vi "Encoder_sub_VI.vi"(8 "error in (no error)":errorcluster) -> (0 "error out":errorcluster, 3 "Encoder Output":T1)   [LabVIEW 2017]
uses:
  Encoder Cluster.ctl
  <vilib>/myRIO/Common/Instrument Driver Framework/myRIO v1.0/Encoder/typedefs/Encoder Count Direction Enum.ctl
  <vilib>/myRIO/Common/Instrument Driver Framework/myRIO v1.0/Encoder/typedefs/Encoder Signal Mode.ctl
  <vilib>/myRIO/Instrument Drivers/Onboard IO/Encoder/typedefs/Encoder Reference.ctl
  <vilib>/myRIO/Common/Instrument Driver Framework/Utilities/typedefs/myRIO Generic Hardware Reference.ctl
  <vilib>/myRIO/Common/Instrument Driver Framework/Utilities/typedefs/Hardware Version Enum.ctl
  <vilib>/myRIO/Common/Instrument Driver Framework/Utilities/typedefs/myRIO v1.0 Reference.ctl
  <vilib>/myRIO/Common/Instrument Driver Framework/Utilities/typedefs/Generic FPGA Reference.ctl
  <vilib>/myRIO/Common/Instrument Driver Framework/myRIO v1.0/Encoder/typedefs/Encoder Channels Enum.ctl
  <vilib>/myRIO/Common/Instrument Driver Framework/myRIO v1.0/Encoder/typedefs/Encoder Configuration v1.0.ctl
  <vilib>/userdefined/High Color/nirio_resource_hc.ctl
  <vilib>/myRIO/Common/Instrument Driver Framework/Utilities/vis/Is FPGA Ref Available.vi
  <vilib>/myRIO/Common/Instrument Driver Framework/myRIO v1.0/Encoder/vis/myRIO v1.1 Open Encoder.vi
  <vilib>/myRIO/Instrument Drivers/Onboard IO/Encoder/vis/Read.vi
  <vilib>/myRIO/Common/Instrument Driver Framework/Utilities/vis/Validate Channels.vi
  <vilib>/myRIO/Common/Instrument Driver Framework/myRIO v1.0/Encoder/vis/myRIO v1.0 Reserve Encoder.vi
  <vilib>/myRIO/Common/Instrument Driver Framework/myRIO v1.0/Encoder/vis/myRIO v1.0 Build MUX Configuration Encoder.vi
  <vilib>/myRIO/Common/Instrument Driver Framework/myRIO v1.0/Resource Manager/vis/myRIO v1.0 Reserve Channel List.vi
  <vilib>/myRIO/Common/Instrument Driver Framework/myRIO v1.0/Resource Manager/vis/myRIO v1.0 Create Configuration List.vi
  <vilib>/myRIO/Common/Instrument Driver Framework/myRIO v1.0/Resource Manager/vis/myRIO v1.0 Reserve Channel.vi
  <vilib>/myRIO/Common/Instrument Driver Framework/myRIO v1.0/Resource Manager/vis/myRIO v1.0 Unreserve Channel.vi
  <vilib>/myRIO/Common/Instrument Driver Framework/myRIO v1.0/Resource Manager/vis/myRIO v1.0 Build Mutex Name.vi
  <vilib>/Utility/VariantDataType/GetNumericInfo.vi
  <vilib>/Utility/error.llb/Error Cluster From Error Code.vi
  <vilib>/myRIO/Common/Instrument Driver Framework/myRIO v1.0/myRIO v1.1 Open.vi
  <vilib>/myRIO/Common/Instrument Driver Framework/Utilities/vis/IO Manager.vi
  <vilib>/myRIO/Common/Instrument Driver Framework/Utilities/vis/Configuration Manager.vi
  <vilib>/myRIO/Common/Instrument Driver Framework/myRIO v1.0/Resource Manager/vis/myRIO v1.0 Configure IO.vi
  <vilib>/myRIO/Common/Instrument Driver Framework/myRIO v1.0/myRIO v1.0 Close.vi
  <vilib>/myRIO/Common/Instrument Driver Framework/myRIO v1.0/Encoder/vis/myRIO v1.0 Configure Encoder.vi
  <vilib>/myRIO/Common/Instrument Driver Framework/myRIO v1.0/Encoder/vis/myRIO v1.0 Read Encoder.vi
  <vilib>/myRIO/Express VI/Onboard IO/Encoder/Encoder Express VI.xnode
  <vilib>/myRIO/Instrument Drivers/Onboard IO/Encoder/vis/myRIO Encoder Open.xnode
  <vilib>/myRIO/Instrument Drivers/Onboard IO/Encoder/Encoder.lvlib
panel:
  in  "Reset Y Counter":bool
  in  "Reset X Counter":bool
  in  "Encoder Input":T1
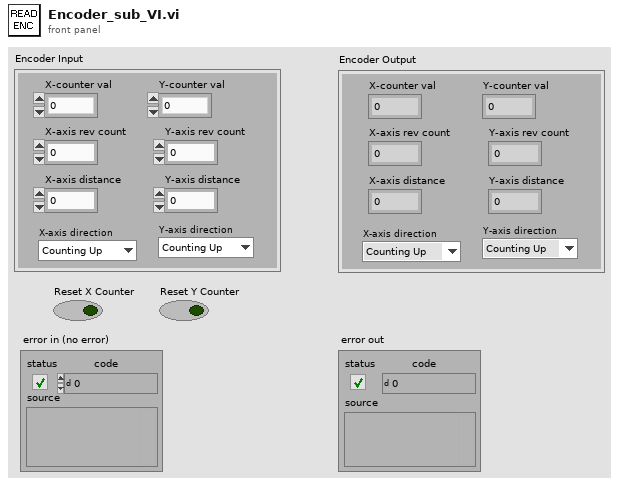
[diagram p1: front panel]
types:
  T1 = typedef "Encoder Cluster.ctl" = cluster{"Y-axis rev count":dbl, "Y-axis distance":dbl, "X-axis rev count":dbl, "X-axis distance":dbl, "Y-axis direction":T2, "X-axis direction":T2, "X-counter val":i32, "Y-counter val":i32}
  T2 = typedef "Encoder Count Direction Enum.ctl" = enum16{"Counting Up", "Counting Down"}
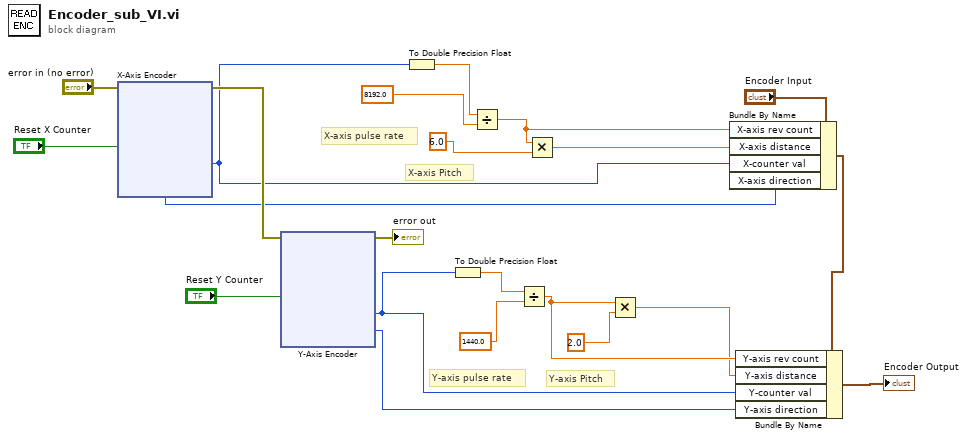
[diagram p0: block diagram]
diagram:
  # "Y-axis Pitch"
  # "Y-axis pulse rate"
  # "X-axis pulse rate"
  # "X-axis Pitch"
  n1 = xnode "X-Axis Encoder"("Reset Counter"="Reset X Counter", "error in (no error)"="error in (no error)") -> ("Counter Value"=w3:i32, "Counter Direction"=w4:T2, "error out"=w19:errorcluster)  [unwired: 1 out]
  n2 = xnode "Y-Axis Encoder"("Reset Counter"="Reset Y Counter", "error in (no error)"=w19) -> ("Counter Value"=w7:i32, "Counter Direction"=w6:T2, "error out"=→"error out":errorcluster)  [unwired: 1 out]
  n3 = To Double Precision Float(number=w3) -> (double precision float=w14:dbl)
  n4 = To Double Precision Float(number=w7) -> (double precision float=w15:dbl)
  n5 = Divide(x=w14, y=8192.0) -> (x/y=w13:dbl)
  n6 = Divide(x=w15, y=1440.0) -> (x/y=w5:dbl)
  n7 = Multiply(x=w13, y=6.0) -> (x*y=w2:dbl)
  n8 = Multiply(x=w5, y=2.0) -> (x*y=w1:dbl)
  n9 = Bundle By Name(cluster="Encoder Input", "X-axis rev count"=w13, "X-axis distance"=w2, "X-counter val"=w3, "X-axis direction"=w4) -> (w8:T1)
  n10 = Bundle By Name(cluster=w8, "Y-axis rev count"=w5, "Y-axis distance"=w1, "Y-counter val"=w7, "Y-axis direction"=w6) -> (→"Encoder Output":T1)
